vi "CalcAngleError.vi"(9 "DesiredAngle":dbl format="%#_13g", 10 "ActualAngle":dbl format="%#_13g") -> (2 "Error":dbl)   [LabVIEW 2013]
doc: "Calculates the difference between the actual angle and the desired angle. The returned error is on the interval [-180, 180]. (A positive number means the robot must rotate counterclockwise, a negative number means the robot must rotate clockwise.)"
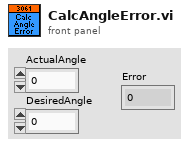
[diagram p1: front panel]
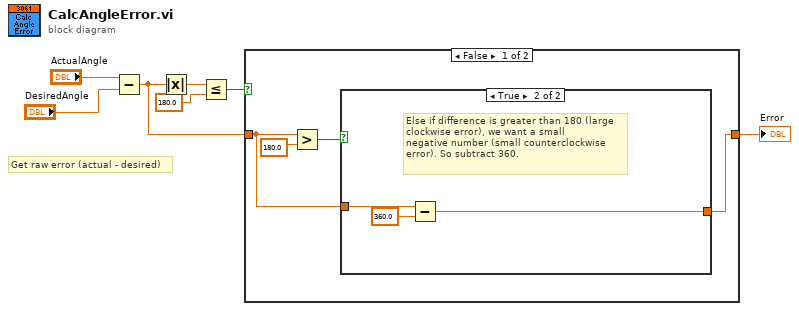
[diagram p0: block diagram]
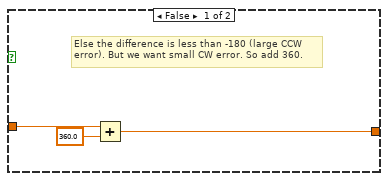
[diagram p2: hidden frame]
diagram:
  # "Get raw error (actual - desired)"
  n1 = Subtract(x="ActualAngle", y="DesiredAngle") -> (x-y=w4:dbl)
  n2 = Absolute Value(x=w4) -> (abs(x)=w7:dbl)
  n3 = Less Or Equal?(x=w7, y=180.0) -> (x <= y?=w5:bool)
  n4 = case shown="False" w5 {
    tunnel: w4 -> [w10 w18]
    tunnel: [w8 w18] -> w3
    frame False {
      n5 = Greater?(x=w10, y=180.0) -> (0:w9:bool)
      n6 = case shown="True" w9 {
        tunnel: w10 -> [w14 w17]
        tunnel: [w12 w15] -> w8
        frame False {
          # "Else the difference is less than -180 (large CCW\nerror). But we want small CW error. So add 360."
          n7 = Add(x=w14, y=360.0) -> (x+y=w12:dbl)
        }
        frame True {
          # "Else if difference is greater than 180 (large\nclockwise error), we want a small\nnegative number (small counterclockwise\nerror). So subtract 360."
          n8 = Subtract(x=w17, y=360.0) -> (x-y=w15:dbl)
        }
      }
    }
    frame True {
      # "If magnitude of difference is less than 180, no processing needed"
    }
  }
  "Error" <- w3
